vi "Create.vi"(2 "Plots":i32) -> (14 "Data":cluster{cluster{dbl, dbl}[]}[](array[cluster]))   [LabVIEW 2018]
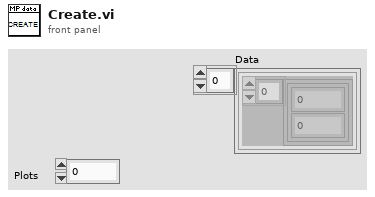
[diagram p1: front panel]
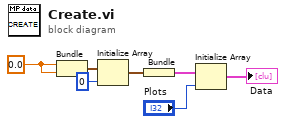
[diagram p0: block diagram]
diagram:
  w7 = 0.0
  n1 = Bundle(w7, w7) -> (w6:cluster{dbl, dbl})  [unwired: 1 in]
  n2 = Initialize Array(w6, 0 ("dimension size")) -> (w4:cluster{dbl, dbl}[])
  n3 = Bundle(w4) -> (w3:cluster{cluster{dbl, dbl}[]})  [unwired: 1 in]
  n4 = Initialize Array(w3, "Plots") -> (→"Data":cluster{cluster{dbl, dbl}[]}[])
